vi "test RT Start.vi"(8 "error in (no error)":errorcluster, 11 "RT Start in":refnum<class "RT Start.lvclass">) -> (0 "error out":errorcluster, 3 "RT Start out":refnum<class "RT Start.lvclass">)   [LabVIEW 2016, in "RT Start.lvclass"]
uses:
  RT Start.lvclass
  1553 Board/1553 Board.lvclass
  PPLs/FPGA Interface.lvlibp/FPGA Interface/FPGA Interface.lvclass
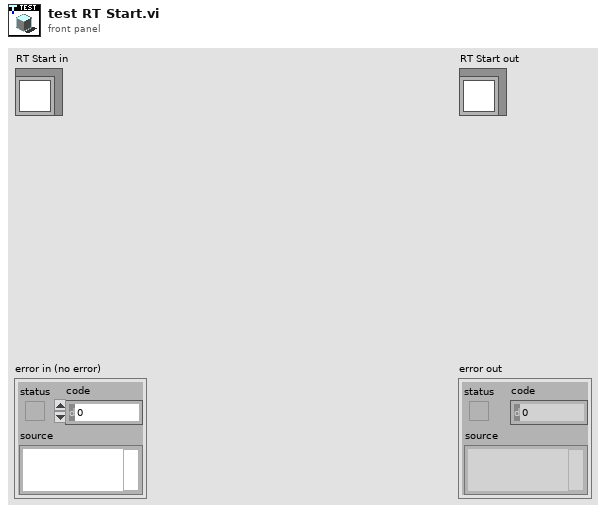
[diagram p1: front panel]
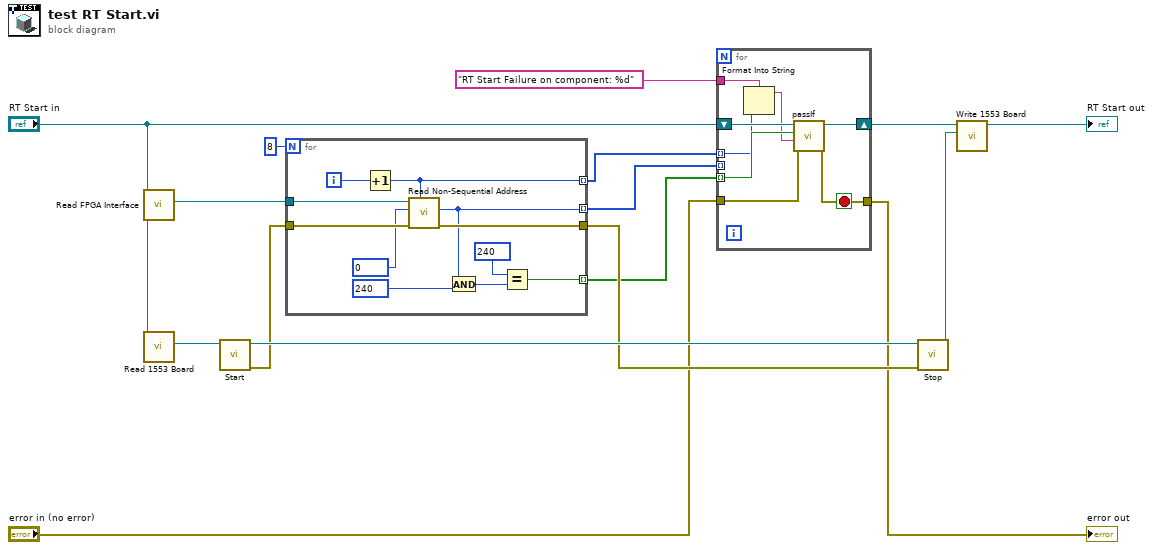
[diagram p0: block diagram]
diagram:
  n1 = call-dynamic "Read FPGA Interface.vi"("1553 Test in"="RT Start in") -> ("FPGA Interface"=w12:refnum<class "FPGA Interface.lvclass">)  [unwired: 8 in, 2 out]
  n2 = call-dynamic "Read 1553 Board.vi"("1553 Test in"="RT Start in") -> ("1553 Board"=w16:refnum<class "1553 Board.lvclass">)  [unwired: 8 in, 2 out]
  n3 = call-dynamic "Start.vi"("1553 Board in"=w16) -> ("error out"=w10:errorcluster, "1553 Board out"=w13:refnum<class "1553 Board.lvclass">)  [unwired: 9 in]
  n4 = for {
    N: 8 -> [_]
    tunnel: w12 -> [w27]
    tunnel: w10 -> [w25]
    tunnel: [w20] -> w4 mode=indexing
    tunnel: [w19] -> w3 mode=indexing
    tunnel: [w18] -> w9
    tunnel: [w17] -> w1 mode=indexing
    i -> [w26]
    n5 = Increment(x=w26) -> (x+1=w19:i32)
    n6 = call-dynamic "Read Non-Sequential Address.vi"("Target IC (1-8)"=w19, "error in (no error)"=w25, "Address"=u16 0, "FPGA Interface in"=w27) -> ("error out"=w18:errorcluster, "Data"=w17:u16)  [unwired: 6 in]
    n7 = And(x=w17, y=u16 240) -> (x .and. y?=w21:u16)
    n8 = Equal?(x=u16 240, y=w21) -> (x = y?=w20:bool)
  }
  n9 = for {
    shift-right: [w34] -> w7
    shift-left: "RT Start in" -> [w35]
    tunnel: "error in (no error)" -> [w33]
    tunnel: [w32] -> w5
    tunnel: w4 -> [w31] mode=indexing
    tunnel: w3 -> [w29] mode=indexing
    tunnel: "RT Start Failure on component: %d" ("custom report message (\"\")") -> [w30]
    tunnel: w1 -> [_] mode=indexing
    stop <- w32 stop-if-true
    n10 = Format Into String(format string=w30, w29) -> (resulting string=w28:string)  [unwired: 2 in, 1 out]
    n11 = call-dynamic "passIf.vi"("error in (no error)"=w33, "message (\"\")"=w28, "pass"=w31, "TestCase in"=w35) -> ("error out"=w32:errorcluster, "TestCase out"=w34:refnum<class "RT Start.lvclass">)  [unwired: 6 in]
  }
  "error out" <- w5
  n12 = call-dynamic "Stop.vi"("error in (no error)"=w9, "1553 Board in"=w13) -> ("1553 Board out"=w14:refnum<class "1553 Board.lvclass">)  [unwired: 8 in, 1 out]
  n13 = call-dynamic "Write 1553 Board.vi"("1553 Board"=w14, "1553 Test in"=w7) -> ("1553 Test out"=→"RT Start out":refnum<class "RT Start.lvclass">)  [unwired: 8 in, 1 out]
